vi "Sort Unwired Terminals.vi"(8 "error in (no error)":errorcluster, 11 "Terms in":refnum<vi>[](array[refnum])) -> (0 "error out":errorcluster, 2 "Unwired Sink Terms":refnum<vi>[](array[refnum]), 3 "Unwired Source Terms":refnum<vi>[](array[refnum]))   [LabVIEW 2016]
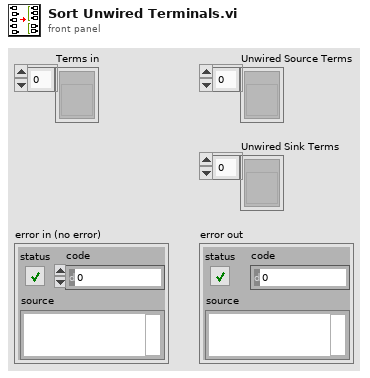
[diagram p1: front panel]
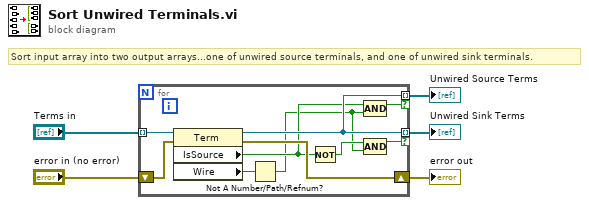
[diagram p0: block diagram]
diagram:
  # "Sort input array into two output arrays...one of unwired source terminals, and one of unwired sink terminals."
  n1 = for {
    shift-right: [w13] -> w3
    shift-left: "error in (no error)" -> [w14]
    tunnel: "Terms in" -> [w15] mode=indexing
    tunnel: [w12] -> w2 mode=indexing if=w8
    tunnel: [w12] -> w1 mode=indexing if=w9
    n2 = property class="Term"(reference=w15, error in=w14) -> (reference out=w12:refnum<vi>, error out=w13:errorcluster, "IsSource"=w11:bool, "Wire"=w10:refnum<vi>)
    n3 = Not A Number/Path/Refnum?(number/path/refnum=w10) -> (NaN/Path/Refnum?=w6:bool)
    n4 = Not(x=w11) -> (.not. x?=w7:bool)
    n5 = Compound Arithmetic op=AND(w11, w6) -> (w9:bool)
    n6 = Compound Arithmetic op=AND(w7, w6) -> (w8:bool)
  }
  "error out" <- w3
  "Unwired Sink Terms" <- w2
  "Unwired Source Terms" <- w1
